vi "Main.vi"() -> ()   [LabVIEW 2017]
uses:
  LabVIEW/Controls/Recording Settings.ctl
  LabVIEW/Controls/Probe Dimensions.ctl
  LabVIEW/Controls/Rigid Body Info.ctl
  LabVIEW/Controls/Position.ctl
  LabVIEW/Controls/Orientation.ctl
  LabVIEW/Controls/Room Dimensions.ctl
  LabVIEW/Controls/Refnums.ctl
  <vilib>/userdefined/High Color/IMAQdx.ctl
  LabVIEW/Controls/Tracker Type.ctl
  LabVIEW/Controls/COM Port.ctl
  LabVIEW/Controls/Frame Grabber State.ctl
  LabVIEW/Controls/Optitrack State.ctl
  LabVIEW/Controls/Enabled State Control.ctl
  LabVIEW/Controls/Frame Grabber Data.ctl
  <vilib>/vision/Image Controls.llb/IMAQ Image.ctl
  <vilib>/vision/Avi.llb/IMAQ AVI2 Refnum.ctl
panel:
  out "Time (s)":dbl
  in  "Gestation":string
  in  "Connection Settings":T4={"Frame Grabber"="cam1", "Tracker"=enum."Aurora", "Port"=enum."COM1"} caption="These settings must be set BEFORE running the program!"
  in  "Refnums":T5
  out "Tracked?":bool
  out "Crop ROI":i32[](array[numeric])
  in  "Clear Crop":bool
  in  "Append":bool
  in  "Presentation":string
  in  "Crop":bool
  in  "Pause":bool
  out "Video Playback Filename":path
  in  "Frame Slider":u32(slide) scale=0.0..1138.0
  in  "Playback":bool
  in  "Room Dimensions":T6={"Room Width"=1000.0, "Room Depth"=1000.0, "Room Height"=1000.0}
  in  "Home":bool
  in  "Probe Dimensions":T7={"Probe Width"=50.0, "Probe Depth"=75.0, "Probe Height"=100.0} {"Probe Height" min=0.001; "Probe Depth" min=0.001; "Probe Width" min=0.001}
  in  "Recording Settings":T8={"Folder to Save Recording"=path "C:/Users/lydia/Desktop/Images", "Recording Name"="Test", "Video FPS"=5.0, "Codec"=3, "Operator"=0, "Tracker FPS"=40.0} {"Tracker FPS" min=1.0 max=100.0 format="%_6g"; "Operator" items=["Novice", "Expert"]; "Codec" items=["Cinepak Codec by Radius", "Intel IYUV codec", "Microsoft Video 1", "FF Video Codec 1 (FFV1) (NI Vision)", "Motion JPEG (NI Vision)", "Y800 Uncompressed Grey Scale (NI Vision)", "YUV 4:2:0 Planar (NI Vision)"]; "Video FPS" min=0.01 max=100.0 format="%.4f"}
  in  "Record":bool
  out "Tracker \nConnected?":bool
  out "Frame Grabber \nConnected?":bool
  out "Ultrasound Image":T9(plugin-control)
  in  "Live":bool
  in  "stop":bool
  in  "Probe Position":enum32{"3D", "Data"}(tab)
  out "Probe Position":refnum<vi>(3d-picture)
  out "Rigid Body":T10 caption="Probe Position Data"
  # "Frame"
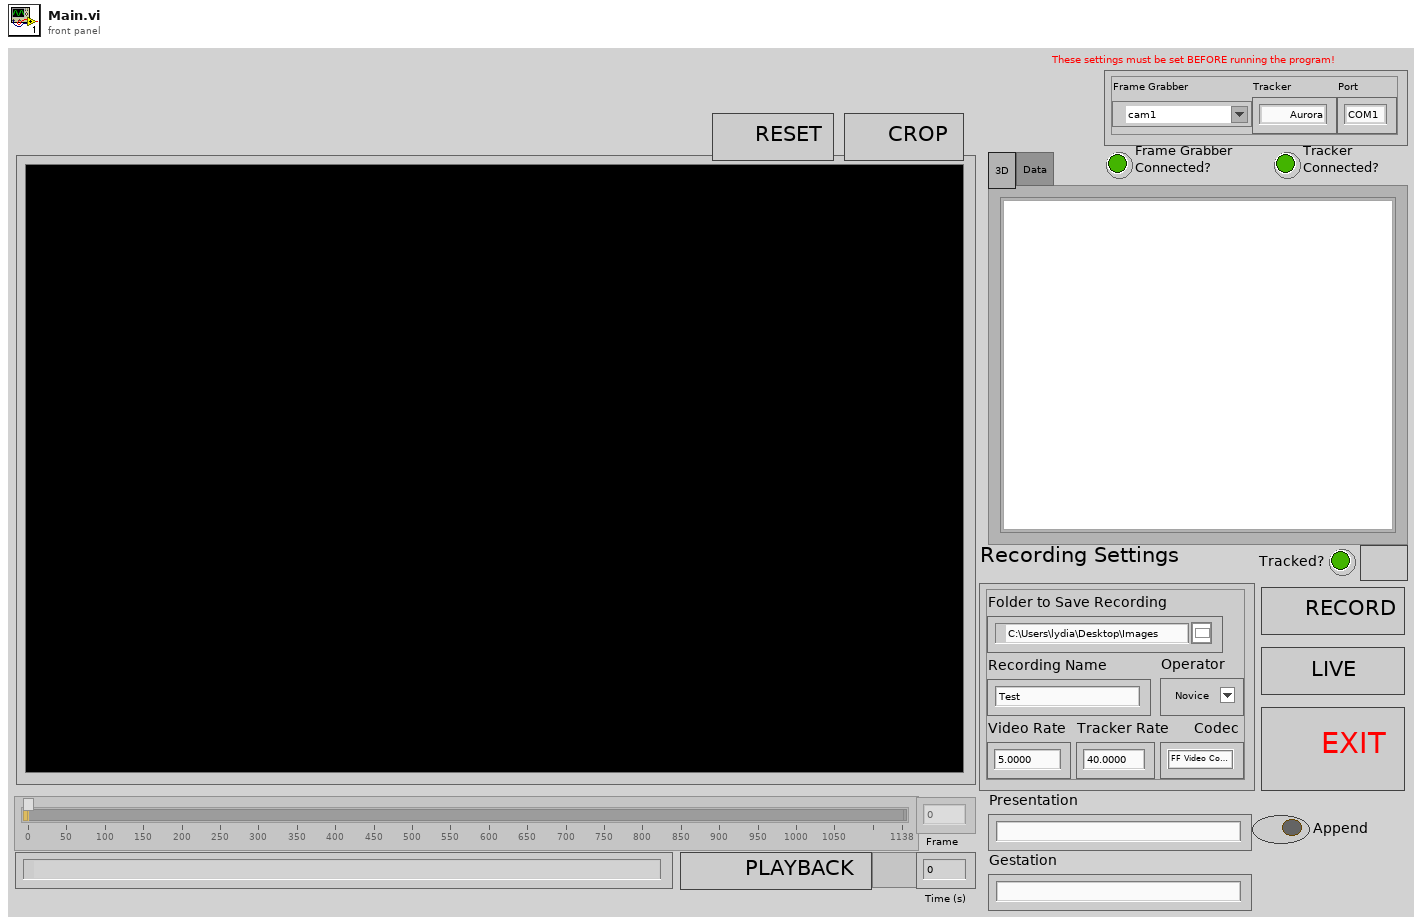
[diagram p1: front panel]
types:
  T1 = typedef "IMAQdx.ctl" = refnum<k21>
  T2 = typedef "Tracker Type.ctl" = enum16{"Aurora", "OptiTrack"}
  T3 = typedef "COM Port.ctl" = enum16{"COM1", "COM2", "COM3", "COM4", "COM5", "COM6", "COM7", "COM8", "COM9"}
  T4 = cluster{"Frame Grabber":T1, "Tracker":T2, "Port":T3}
  T5 = typedef "Refnums.ctl" = cluster{"Live Refnum":refnum<vi>, "Record Refnum":refnum<vi>, "Recording Settings Refnum":refnum<vi>, "Playback Refnum":refnum<vi>, "Frame Slider Refnum":refnum<vi>, "Pause Refnum":refnum<vi>, "Home Refnum":refnum<vi>, "Crop Refnum":refnum<vi>, "Clear Crop Refnum":refnum<vi>, "Connection Settings Refnum":refnum<vi>, "stop refnum":refnum<vi>}
  T6 = typedef "Room Dimensions.ctl" = cluster{"Room Width":dbl, "Room Depth":dbl, "Room Height":dbl}
  T7 = typedef "Probe Dimensions.ctl" = cluster{"Probe Width":sgl, "Probe Depth":sgl, "Probe Height":sgl}
  T8 = typedef "Recording Settings.ctl" = cluster{"Folder to Save Recording":path, "Recording Name":string, "Video FPS":dbl, "Codec":u16, "Operator":u16, "Tracker FPS":dbl}
  T9 = typedef "IMAQ Image.ctl" = refnum<image>
  T10 = typedef "Rigid Body Info.ctl" = cluster{"Position":T11, "Orientation":T12, "Quaternion":cluster{"qx":sgl, "qy":sgl, "qz":sgl, "qw":sgl}, "Tracked?":bool}
  T11 = typedef "Position.ctl" = cluster{"x (mm)":sgl, "y (mm)":sgl, "z (mm)":sgl}
  T12 = typedef "Orientation.ctl" = cluster{"Pitch (rad)":sgl, "Yaw (rad)":sgl, "Roll (rad)":sgl}
  T13 = typedef "Enabled State Control.ctl" = enum16{"Wait", "Start Live", "Start Recording", "Start Playback", "Shutdown"}
  T14 = typedef "Optitrack State.ctl" = enum16{"Wait", "Init", "Grab Rigid Body Data", "Error Handling", "Shutdown"}
  T15 = typedef "Frame Grabber State.ctl" = enum16{"Wait", "Init", "Update Geometry", "Set Crop ROI", "Clear Crop ROI", "Configure Live", "Configure Recording", "Start Playback", "Grab Live Frame", "Record Frame", "Playback Frame", "Unconfigure Live", "End Recording", "Stop Playback", "Error Handling", "Shutdown"}
  T16 = typedef "Queues.ctl" = cluster{"Frame Grabber State":refnum<queue>, "Tracker State":refnum<queue>}
  T17 = typedef "Frame Grabber Data.ctl" = cluster{"Camera Session":T1, "Frame":T9, "AVI Refnum":T18, "Codecs":string[], "Frame number":u32, "Tracking File Refnum":refnum<file>, "Tick Count":u32, "Probe Object":refnum<vi>, "Playback Probe Data":dbl[][], "Rigid Body":T10, "Total no frames playback":u32, "Playback Video FPS":u32, "Camera connected?":bool, "Scene":refnum<vi>, "Frame Number Refnum":refnum<vi>, "Cropped Frame":T9, "Playback Tracker FPS":u32, "Crop ROI":i32[], "Presentation Values":string[], "Elapsed time (ms)":u32, "Camera frames playback":u32, "Gestation":string}
  T18 = typedef "IMAQ AVI2 Refnum.ctl" = refnum<k20>
  T19 = enum8{"Enabled", "Disabled", "Disabled and Grayed Out"}
  T20 = typedef "Tracking Data.ctl" = cluster{"VISA resource name":refnum<visa-resource-name>, "Packet Data":T21, "Rigid Body Data":T10, "Position Array":dbl[][], "Tracker":T2}
  T21 = typedef "Packet Data.ctl" = cluster{"Frame Number (UINT32)":u32, "Number of Rigid Bodies (UINT32)":u32, "Timestamp (double float)":dbl}
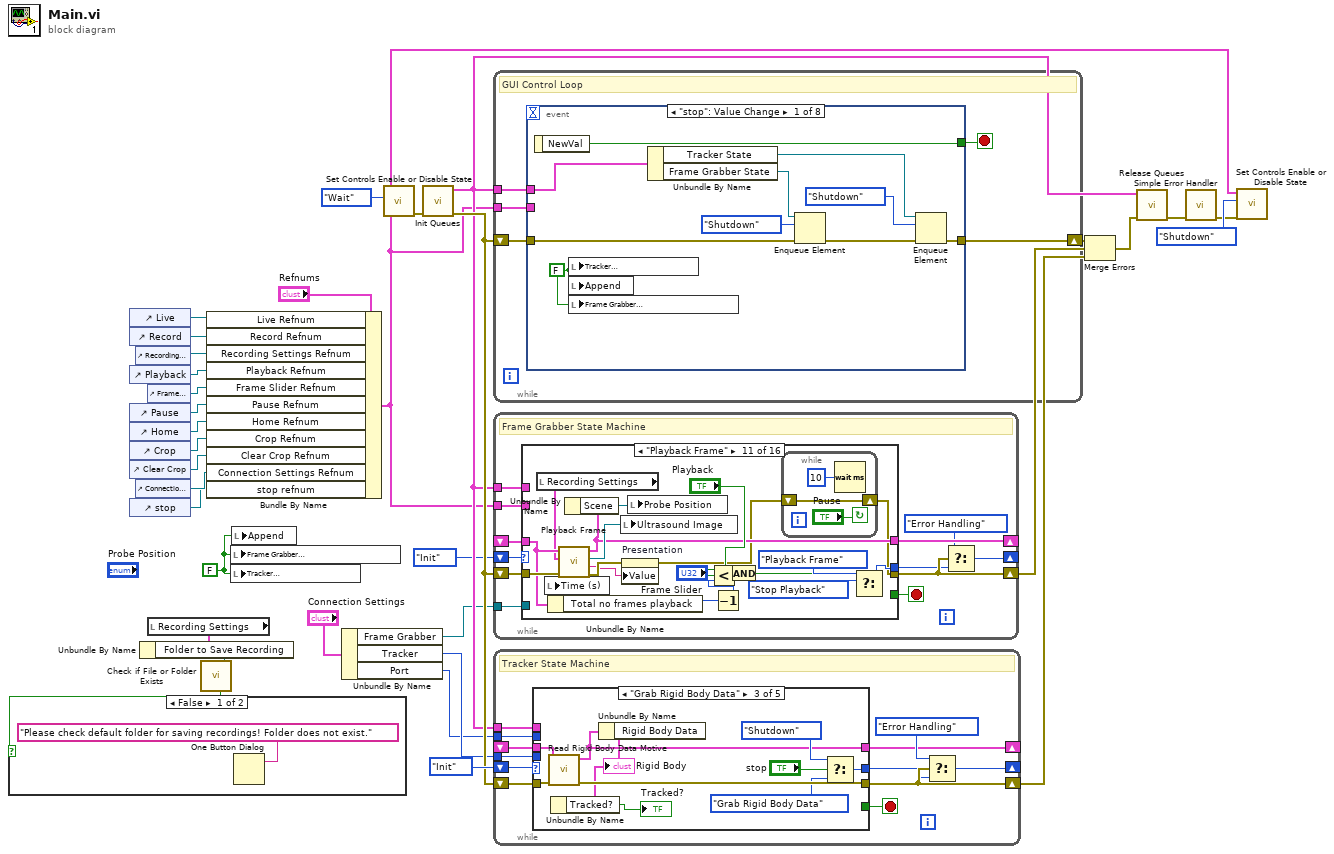
[diagram p0: block diagram]
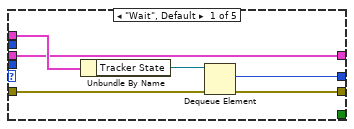
[diagram p3: hidden frame]
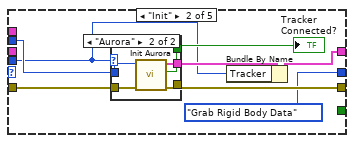
[diagram p4: hidden frame]
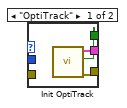
[diagram p5: hidden frame]
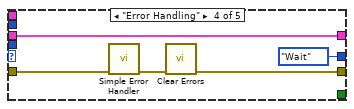
[diagram p6: hidden frame]
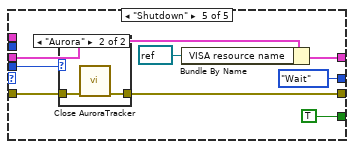
[diagram p7: hidden frame]
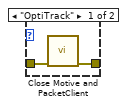
[diagram p8: hidden frame]
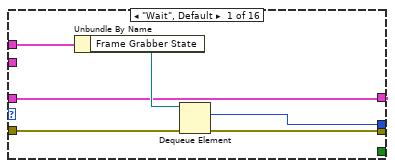
[diagram p9: hidden frame]
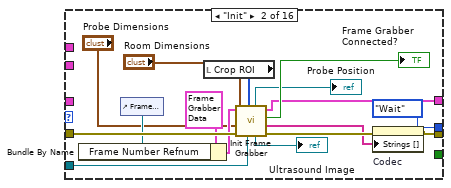
[diagram p10: hidden frame]
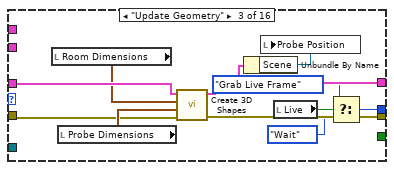
[diagram p11: hidden frame]
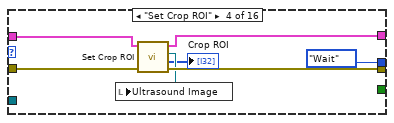
[diagram p12: hidden frame]
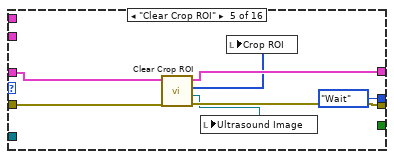
[diagram p13: hidden frame]
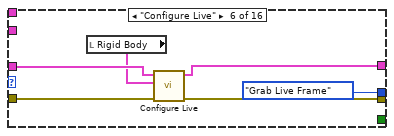
[diagram p14: hidden frame]
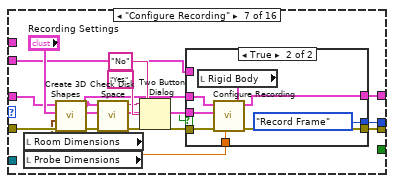
[diagram p15: hidden frame]
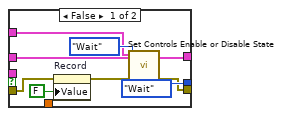
[diagram p16: hidden frame]
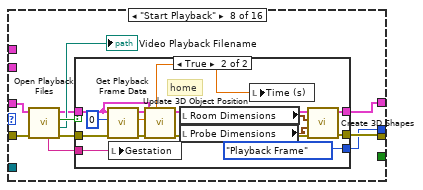
[diagram p17: hidden frame]
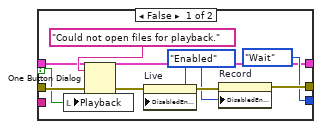
[diagram p18: hidden frame]
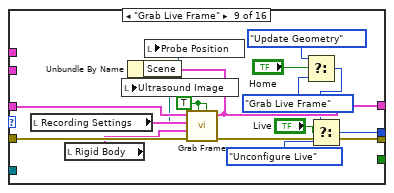
[diagram p19: hidden frame]
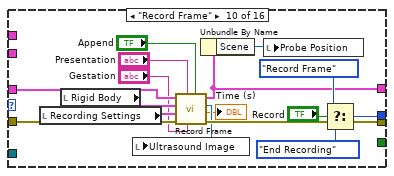
[diagram p20: hidden frame]
diagram:
  w13 = FALSE ("Camera Connected?")
  n1 = control-ref of="Live"() -> (w25:refnum<vi>)
  n2 = control-ref of="Record"() -> (w24:refnum<vi>)
  n3 = control-ref of="Playback"() -> (w22:refnum<vi>)
  n4 = control-ref of="Pause"() -> (w20:refnum<vi>)
  n5 = control-ref of="Home"() -> (w19:refnum<vi>)
  n6 = control-ref of="Crop"() -> (w18:refnum<vi>)
  n7 = control-ref of="Clear Crop"() -> (w17:refnum<vi>)
  n8 = control-ref of="stop"() -> (w1:refnum<vi>)
  n9 = control-ref of="Recording Settings"() -> (w23:refnum<vi>)
  n10 = control-ref of="Connection Settings"() -> (w2:refnum<vi>)
  n11 = control-ref of="Frame Slider"() -> (w21:refnum<vi>)
  n12 = local read "Recording Settings"() -> (w12:T8)
  n13 = Unbundle By Name(w12) -> ("Folder to Save Recording"=w11:path)
  n14 = call <vilib>:"Check if File or Folder Exists.vi"("path"=w11) -> ("file or folder exists?"=w10:bool)  [unwired: 8 in, 2 out]
  n15 = case shown="False" w10 {
    frame False {
      n16 = One Button Dialog(message="Please check default folder for saving recordings! Folder does not exist.") -> ()  [unwired: 1 in, 1 out]
    }
    frame True {
    }
  }
  n17 = Bundle By Name(cluster="Refnums", "Live Refnum"=w25, "Record Refnum"=w24, "Recording Settings Refnum"=w23, "Playback Refnum"=w22, "Frame Slider Refnum"=w21, "Pause Refnum"=w20, "Home Refnum"=w19, "Crop Refnum"=w18, "Clear Crop Refnum"=w17, "Connection Settings Refnum"=w2, "stop refnum"=w1) -> (w7:T5)
  n18 = local write "Frame Grabber \nConnected?"(w13) -> ()
  n19 = local write "Tracker \nConnected?"(w13) -> ()
  n20 = local write "Append"(w13) -> ()
  n21 = Unbundle By Name("Connection Settings") -> ("Frame Grabber"=w5:T1, "Tracker"=w4:T2, "Port"=w3:T3)
  n22 = call "Set Controls Enable or Disable State.vi"("Refnum State"=Enabled_State_Control."Wait", "Refnums In"=w7) -> ("error out"=w15:errorcluster)  [unwired: 9 in]
  n23 = call "Init Queues.vi"("error in (no error) in"=w15) -> ("error out"=w29:errorcluster, "Queues"=w28:T16)  [unwired: 9 in]
  n24 = while {
    shift-right: [w38] -> w34
    shift-left: w29 -> [w39]
    tunnel: w28 -> [w37]
    tunnel: w7 -> [w36]
    stop <- w40 stop-if-true
    # "GUI Control Loop"
    n25 = event shown="[0] \"stop\": Value Change" {
      selector: _ -> [_ _ _ _ _ _ _ _]
      dyn-events: _ -> [_ _ _ _ _ _ _ _]
      timeout: _ -> [_ _ _ _ _ _ _ _]
      tunnel: [w43 _ _ _ _ _ _ _] -> w40
      tunnel: w39 -> [w42 w63 w77 w79 w87 w92 w105 w106]
      tunnel: [w46 w56 w68 w78 w83 w88 w96 w106] -> w38
      tunnel: w37 -> [w50 w60 w74 w82 w86 w91 w102 _]
      tunnel: w36 -> [_ w55 w70 _ _ _ w98 _]
      event "stop": Value Change {
        w41 = FALSE ("Run")
        n26 = event-data() -> ("NewVal"=w43:bool)  [unwired: 1 in]
        n27 = local write "Tracker \nConnected?"(w41) -> ()
        n28 = local write "Append"(w41) -> ()
        n29 = local write "Frame Grabber \nConnected?"(w41) -> ()
        n30 = Unbundle By Name(w50) -> ("Tracker State"=w45:refnum<queue>, "Frame Grabber State"=w49:refnum<queue>)
        n31 = Enqueue Element(queue=w49, element=Frame_Grabber_State."Shutdown", error in (no error)=w42) -> (error out=w47:errorcluster)  [unwired: 1 in, 2 out]
        n32 = Enqueue Element(queue=w45, element=Optitrack_State."Shutdown", error in (no error)=w47) -> (error out=w46:errorcluster)  [unwired: 1 in, 2 out]
      }
      event "Live": Value Change {
        n33 = event-data() -> ("NewVal"=w52:bool)  [unwired: 1 in]
        n34 = Unbundle By Name(w60) -> ("Frame Grabber State"=w59:refnum<queue>)
        n35 = Select(t=Frame_Grabber_State."Configure Live", s=w52, f=Frame_Grabber_State."Wait") -> (s? t:f=w61:T15)
        n36 = Enqueue Element(queue=w59, element=w61, error in (no error)=w63) -> (error out=w57:errorcluster)  [unwired: 1 in, 2 out]
        n37 = Select(t=Enabled_State_Control."Start Live" ("Refnum State"), s=w52, f=Enabled_State_Control."Wait") -> (s? t:f=w53:T13)
        n38 = call "Set Controls Enable or Disable State.vi"("error in (no error)"=w57, "Refnum State"=w53, "Refnums In"=w55) -> ("error out"=w56:errorcluster)  [unwired: 8 in]
      }
      event "Playback": Value Change {
        n39 = event-data() -> ("NewVal"=w66:bool)  [unwired: 1 in]
        n40 = Unbundle By Name(w74) -> ("Frame Grabber State"=w73:refnum<queue>)
        n41 = Select(t=Frame_Grabber_State."Start Playback", s=w66, f=Frame_Grabber_State."Wait") -> (s? t:f=w75:T15)
        n42 = Enqueue Element(queue=w73, element=w75, error in (no error)=w77) -> (error out=w69:errorcluster)  [unwired: 1 in, 2 out]
        n43 = Select(t=Enabled_State_Control."Start Playback", s=w66, f=Enabled_State_Control."Wait" ("Refnum State")) -> (s? t:f=w65:T13)
        n44 = local write "Pause"(FALSE ("Pause")) -> ()
        n45 = call "Set Controls Enable or Disable State.vi"("error in (no error)"=w69, "Refnum State"=w65, "Refnums In"=w70) -> ("error out"=w68:errorcluster)  [unwired: 8 in]
      }
      event "Home": Value Change {
        n46 = event-data() -> ()  [unwired: 1 in, 4 out]
        n47 = Unbundle By Name(w82) -> ("Frame Grabber State"=w81:refnum<queue>)
        n48 = Enqueue Element(queue=w81, element=Frame_Grabber_State."Update Geometry", error in (no error)=w79) -> (error out=w78:errorcluster)  [unwired: 1 in, 2 out]
      }
      event "Crop": Value Change {
        n49 = event-data() -> ()  [unwired: 1 in, 4 out]
        n50 = Unbundle By Name(w86) -> ("Frame Grabber State"=w85:refnum<queue>)
        n51 = Enqueue Element(queue=w85, element=Frame_Grabber_State."Set Crop ROI", error in (no error)=w87) -> (error out=w83:errorcluster)  [unwired: 1 in, 2 out]
      }
      event "Clear Crop": Value Change {
        n52 = event-data() -> ()  [unwired: 1 in, 4 out]
        n53 = Unbundle By Name(w91) -> ("Frame Grabber State"=w90:refnum<queue>)
        n54 = Enqueue Element(queue=w90, element=Frame_Grabber_State."Clear Crop ROI", error in (no error)=w92) -> (error out=w88:errorcluster)  [unwired: 1 in, 2 out]
      }
      event "Record": Value Change {
        n55 = event-data() -> ("NewVal"=w99:bool)  [unwired: 1 in]
        n56 = Unbundle By Name(w102) -> ("Frame Grabber State"=w101:refnum<queue>)
        n57 = Select(t=Frame_Grabber_State."Configure Recording", s=w99, f=Frame_Grabber_State."Wait") -> (s? t:f=w103:T15)
        n58 = Enqueue Element(queue=w101, element=w103, error in (no error)=w105) -> (error out=w97:errorcluster)  [unwired: 1 in, 2 out]
        n59 = Select(t=Enabled_State_Control."Start Recording" ("Refnum State"), s=w99, f=Enabled_State_Control."Wait" ("Refnum State")) -> (s? t:f=w93:T13)
        n60 = call "Set Controls Enable or Disable State.vi"("error in (no error)"=w97, "Refnum State"=w93, "Refnums In"=w98) -> ("error out"=w96:errorcluster)  [unwired: 8 in]
      }
      event "Presentation": Value Change {
        n61 = event-data() -> ()  [unwired: 1 in, 1 out]
        n62 = local write "Append"(TRUE ("Append")) -> ()
      }
    }
  }
  n63 = while {
    shift-right: [w111] -> _
    shift-left: Frame_Grabber_State."Init" -> [w119]
    shift-right: [w113] -> w33
    shift-left: w29 -> [w118]
    tunnel: w28 -> [w117]
    shift-right: [w115] -> _
    shift-left: _ -> [w114]
    tunnel: w7 -> [w109]
    tunnel: w5 -> [w108]
    stop <- w116 stop-if-true
    # "Frame Grabber State Machine"
    n64 = case shown="\"Playback Frame\"" w119 {
      tunnel: w118 -> [w125 w141 w150 w158 w164 w172 w178 w215 w253 w265 w286 w296 w300 w311 w317 w326]
      tunnel: [w124 w137 w149 w157 w163 w171 w187 w212 w252 w264 w276 w294 w297 w304 w314 w325] -> w113
      tunnel: w117 -> [w123 _ _ _ _ _ _ _ _ _ _ _ _ _ _ _]
      tunnel: [w121 Frame_Grabber_State."Wait" w143 Frame_Grabber_State."Wait" Frame_Grabber_State."Wait" Frame_Grabber_State."Grab Live Frame" w189 w211 w250 w267 w288 Frame_Grabber_State."Wait" Frame_Grabber_State."Wait" Frame_Grabber_State."Wait" Frame_Grabber_State."Wait" Frame_Grabber_State."Wait"] -> w112
      tunnel: [_ _ _ _ _ _ _ _ _ _ _ _ _ _ _ TRUE] -> w116
      tunnel: [w120 w129 w148 w155 w162 w168 w188 w206 w245 w258 w278 w293 w298 w308 w318 w323] -> w115
      tunnel: w114 -> [w120 _ w152 w156 w165 w170 w176 w214 w248 w261 w280 w293 w298 w309 w318 w324]
      tunnel: w109 -> [_ _ _ _ _ _ w179 _ _ _ _ _ _ w301 w313 _]
      tunnel: w108 -> [_ w126 _ _ _ _ _ _ _ _ _ _ _ _ _ _]
      frame "Wait", Default {
        n65 = Unbundle By Name(w123) -> ("Frame Grabber State"=w122:refnum<queue>)
        n66 = Dequeue Element(queue=w122, error in (no error)=w125) -> (element=w121:T15, error out=w124:errorcluster)  [unwired: 1 in, 2 out]
      }
      frame "Init" {
        n67 = control-ref of="Frame Slider"() -> (w134:refnum<vi>)
        n68 = Bundle By Name(cluster=T17 {"Camera Session"="", "Frame"=refnum, "AVI Refnum"=refnum, "Codecs"=[], "Frame number"=0, "Tracking File Refnum"=refnum, "Tick Count"=0, "Probe Object"=refnum, "Playback Probe Data"=[], "Rigid Body"={"Position"={"x (mm)"=0.0, "y (mm)"=0.0, "z (mm)"=0.0}, "Orientation"={"Pitch (rad)"=0.0, "Yaw (rad)"=0.0, "Roll (rad)"=0.0}, "Quaternion"={"qx"=0.0, "qy"=0.0, "qz"=0.0, "qw"=0.0}, "Tracked?"=FALSE}, "Total no frames playback"=0, "Playback Video FPS"=0, "Camera connected?"=FALSE, "Scene"=refnum, "Frame Number Refnum"=refnum, "Cropped Frame"=refnum, "Playback Tracker FPS"=0, "Crop ROI"=[], "Presentation Values"=[], "Elapsed time (ms)"=0, "Camera frames playback"=0, "Gestation"=""} ("Frame Grabber Data"), "Frame Number Refnum"=w134) -> (w133:T17)
        n69 = local read "Crop ROI"() -> (w127:i32[])
        n70 = call "Init Frame Grabber.vi"("Frane Grabber"=w126, "Crop ROI Rectangle"=w127, "Error In"=w141, "Probe Dimensions"="Probe Dimensions", "Room Dimensions"="Room Dimensions", "Frame Grabber Data"=w133) -> ("Error Out"=w138:errorcluster, "Codec Names"=w136:string[], "Frame Grabber Connected?"=→"Frame Grabber \nConnected?":bool, "Frame Grabber Data Out"=w129:T17, "Image Out"=→"Ultrasound Image":T9, "Scene"=→"Probe Position":refnum<vi>)
        n71 = property on="Codec" class="Ring (strict)"(error in=w138, "Strings []"=w136) -> (error out=w137:errorcluster)  [unwired: 1 in, 1 out]
      }
      frame "Update Geometry" {
        n72 = local read "Room Dimensions"() -> (w142:T6)
        n73 = local read "Probe Dimensions"() -> (w151:T7)
        n74 = call "Create 3D Shapes.vi"("error in (no error)"=w150, "Probe Dimensions"=w151, "Room Dimensions"=w142, "Frame Grabber Data In"=w152) -> ("error out"=w149:errorcluster, "Frame Grabber Data Out"=w148:T17)  [unwired: 6 in]
        n75 = Unbundle By Name(w148) -> ("Scene"=w147:refnum<vi>)
        n76 = local write "Probe Position"(w147) -> ()
        n77 = local read "Live"() -> (w146:bool)
        n78 = Select(t=Frame_Grabber_State."Grab Live Frame", s=w146, f=Frame_Grabber_State."Wait") -> (s? t:f=w143:T15)
      }
      frame "Set Crop ROI" {
        n79 = call "Set Crop ROI.vi"("error in (no error)"=w158, "Frame Grabber Data in"=w156) -> ("error out"=w157:errorcluster, "Crop ROI"=→"Crop ROI":i32[], "Image Out"=w154:T9, "Frame Grabber Data out"=w155:T17)  [unwired: 6 in]
        n80 = local write "Ultrasound Image"(w154) -> ()
      }
      frame "Clear Crop ROI" {
        n81 = call "Clear Crop ROI.vi"("error in (no error)"=w164, "Frame Grabber Data in"=w165) -> ("error out"=w163:errorcluster, "Image Out"=w161:T9, "Crop ROI"=w160:i32[], "Frame Grabber Data out"=w162:T17)  [unwired: 6 in]
        n82 = local write "Ultrasound Image"(w161) -> ()
        n83 = local write "Crop ROI"(w160) -> ()
      }
      frame "Configure Live" {
        n84 = local read "Rigid Body"() -> (w167:T10)
        n85 = call "Configure Live.vi"("error in (no error)"=w172, "Rigid Body"=w167, "Frame Grabber Data in"=w170) -> ("error out"=w171:errorcluster, "Frame Grabber Data out"=w168:T17)  [unwired: 7 in]
      }
      frame "Configure Recording" {
        n86 = local read "Room Dimensions"() -> (w173:T6)
        n87 = local read "Probe Dimensions"() -> (w174:T7)
        n88 = call "Create 3D Shapes.vi"("error in (no error)"=w178, "Probe Dimensions"=w174, "Room Dimensions"=w173, "Frame Grabber Data In"=w176) -> ("error out"=w177:errorcluster, "Frame Grabber Data Out"=w175:T17)  [unwired: 6 in]
        n89 = call "Check Disk Space.vi"("Error In"=w177, "Recording Settings"="Recording Settings", "Frame Grabber Data"=w175) -> ("Error Out"=w182:errorcluster, "Max number of frames"=w180:dbl, "Prompt"=w181:string)  [unwired: 5 in, 1 out]
        n90 = Two Button Dialog(message=w181, 1:"No" ("F button name (\"Cancel\")"), 2:"Yes" ("T button name (\"OK\")")) -> (T button?=w183:bool)
        n91 = case shown="True" w183 {
          tunnel: [Frame_Grabber_State."Wait" Frame_Grabber_State."Record Frame"] -> w189
          tunnel: [w197 w204] -> w188
          tunnel: [w192 w203] -> w187
          tunnel: "Recording Settings" -> [_ w201]
          tunnel: w175 -> [w197 w200]
          tunnel: w182 -> [w194 w199]
          tunnel: w180 -> [_ w198]
          tunnel: w179 -> [w190 _]
          frame False {
            n92 = property on="Record" class="Bool (strict)"(error in=w194, "Value"=FALSE ("Record")) -> (error out=w193:errorcluster)  [unwired: 1 in, 1 out]
            n93 = call "Set Controls Enable or Disable State.vi"("error in (no error)"=w193, "Refnum State"=Enabled_State_Control."Wait", "Refnums In"=w190) -> ("error out"=w192:errorcluster)  [unwired: 8 in]
          }
          frame True {
            n94 = local read "Rigid Body"() -> (w202:T10)
            n95 = call "Configure Recording.vi"("Max number of frames"=w198, "error in (no error)"=w199, "Rigid Body"=w202, "Recording Settings"=w201, "Frame Grabber Data In"=w200) -> ("error out"=w203:errorcluster, "Frame Grabber Data Out"=w204:T17)  [unwired: 5 in]
          }
        }
      }
      frame "Start Playback" {
        n96 = call "Open Playback Files.vi"("error in (no error)"=w215, "Frame Grabber Data In"=w214) -> ("error out"=w213:errorcluster, "Playback Video"=→"Video Playback Filename":path, "both exist and open?"=w210:bool, "Frame Grabber Data Out"=w207:T17, "Gestation"=w208:string)  [unwired: 5 in]
        n97 = case shown="True" w210 {
          selector: w210 -> [w217 _]
          tunnel: w213 -> [w221 w235]
          tunnel: [w220 w234] -> w212
          tunnel: [Frame_Grabber_State."Wait" ("f") Frame_Grabber_State."Playback Frame"] -> w211
          tunnel: w208 -> [_ w236]
          tunnel: w207 -> [w216 w228]
          tunnel: [w216 w230] -> w206
          frame False {
            w218 = T19."Enabled" ("Disabled")
            n98 = local write "Playback"(w217) -> ()
            n99 = One Button Dialog(message="Could not open files for playback.") -> ()  [unwired: 1 in, 1 out]
            n100 = property on="Live" class="Bool (strict)"(error in=w221, "DisabledEnum"=w218) -> (error out=w222:errorcluster)  [unwired: 1 in, 1 out]
            n101 = property on="Record" class="Bool (strict)"(error in=w222, "DisabledEnum"=w218) -> (error out=w220:errorcluster)  [unwired: 1 in, 1 out]
          }
          frame True {
            # "home"
            n102 = call "Get Playback Frame Data.vi"("Error In"=w235, "Frame number"=u32 0, "Frame Grabber Data"=w228) -> ("Error Out"=w227:errorcluster, "Time elapsed (s)"=w232:dbl, "New Rigid Body Position"=w229:T10)  [unwired: 4 in, 2 out]
            n103 = local write "Gestation"(w236) -> ()
            n104 = call "Update 3D Object Position.vi"("error in (no error)"=w227, "New Rigid Body Position"=w229, "Frame Grabber Data in"=w228) -> ("error out"=w231:errorcluster, "Frame Grabber Data out"=w226:T17)  [unwired: 7 in]
            n105 = local read "Room Dimensions"() -> (w225:T6)
            n106 = local read "Probe Dimensions"() -> (w224:T7)
            n107 = local write "Time (s)"(w232) -> ()
            n108 = call "Create 3D Shapes.vi"("error in (no error)"=w231, "Probe Dimensions"=w224, "Room Dimensions"=w225, "Frame Grabber Data In"=w226) -> ("error out"=w234:errorcluster, "Frame Grabber Data Out"=w230:T17)  [unwired: 6 in]
          }
        }
      }
      frame "Grab Live Frame" {
        w239 = TRUE
        n109 = local read "Recording Settings"() -> (w249:T8)
        n110 = local read "Rigid Body"() -> (w247:T10)
        n111 = call "Grab Frame.vi"("Live?"=w239, "Grab frame?"=w239, "error in (no error)"=w253, "Rigid Body"=w247, "Recording Settings"=w249, "Frame Grabber Data in"=w248) -> ("error out"=w252:errorcluster, "Frame"=w238:T9, "Frame Grabber Data out"=w245:T17)  [unwired: 2 in, 1 out]
        n112 = local write "Ultrasound Image"(w238) -> ()
        n113 = Unbundle By Name(w245) -> ("Scene"=w246:refnum<vi>)
        n114 = local write "Probe Position"(w246) -> ()
        n115 = Select(t=Frame_Grabber_State."Update Geometry", s="Home", f=Frame_Grabber_State."Grab Live Frame") -> (s? t:f=w241:T15)
        n116 = Select(t=w241, s="Live", f=Frame_Grabber_State."Unconfigure Live") -> (s? t:f=w250:T15)
      }
      frame "Record Frame" {
        n117 = local read "Recording Settings"() -> (w260:T8)
        n118 = local read "Rigid Body"() -> (w263:T10)
        n119 = call "Record Frame.vi"("Append"="Append", "Gestation"="Gestation", "Presentation"="Presentation", "error in (no error)"=w265, "Recording Settings"=w260, "Probe Position"=w263, "Frame Grabber Data In in"=w261) -> ("error out"=w264:errorcluster, "Time elapsed (s)"=→"Time (s)":dbl, "Image"=w262:T9, "Frame Grabber Data out"=w258:T17)  [unwired: 1 in]
        n120 = local write "Ultrasound Image"(w262) -> ()
        n121 = Unbundle By Name(w258) -> ("Scene"=w259:refnum<vi>)
        n122 = local write "Probe Position"(w259) -> ()
        n123 = Select(t=Frame_Grabber_State."Record Frame", s="Record", f=Frame_Grabber_State."End Recording") -> (s? t:f=w267:T15)
      }
      frame "Playback Frame" {
        n124 = local read "Recording Settings"() -> (w277:T8)
        n125 = Unbundle By Name(w280) -> ("Total no frames playback"=w283:u32)
        n126 = call "Playback Frame.vi"("error in (no error)"=w286, "Recording Settings"=w277, "Frame Grabber Data in"=w280) -> ("error out"=w273:errorcluster, "Presentation"=w271:string, "Image"=w285:T9, "Frame Grabber Data out"=w278:T17, "Time elapsed (s)"=w270:dbl)  [unwired: 4 in]
        n127 = local write "Time (s)"(w270) -> ()
        n128 = Unbundle By Name(w278) -> ("Scene"=w275:refnum<vi>)
        n129 = local write "Ultrasound Image"(w285) -> ()
        n130 = property on="Presentation" class="Str"(error in=w273, "Value"=w271) -> (error out=w272:errorcluster)  [unwired: 1 in, 1 out]
        n131 = local write "Probe Position"(w275) -> ()
        n132 = Decrement(x=w283) -> (x-1=w274:u32)
        n133 = Less?(x="Frame Slider", y=w274) -> (x < y?=w284:bool)
        n134 = And(x=w284, y="Playback") -> (x .and. y?=w282:bool)
        n135 = while {
          shift-right: [w290] -> w276
          shift-left: w272 -> [w290]
          stop <- "Pause" continue-if-true
          n136 = Wait (ms)(milliseconds to wait=u32 10) -> ()  [unwired: 1 out]
        }
        n137 = Select(t=Frame_Grabber_State."Playback Frame", s=w282, f=Frame_Grabber_State."Stop Playback") -> (s? t:f=w288:T15)
      }
      frame "Unconfigure Live" {
        n138 = call "Unconfigure Live.vi"("error in (no error)"=w296, "Frame Grabber Data in"=w293) -> ("error out"=w294:errorcluster)  [unwired: 9 in]
      }
      frame "End Recording" {
        n139 = call "End Recording.vi"("error in (no error)"=w300, "Frame Grabber Data in"=w298) -> ("error out"=w297:errorcluster)  [unwired: 9 in]
      }
      frame "Stop Playback" {
        n140 = Unbundle By Name(w309) -> ("AVI Refnum"=w310:T18)
        n141 = call "IMAQ AVI2 Close"("error in (no error)"=w311, "AVI Refnum"=w310) -> ("error out"=w305:errorcluster)  [unwired: 9 in]
        n142 = local write "Playback"(FALSE ("Playback")) -> ()
        n143 = call "Set Controls Enable or Disable State.vi"("error in (no error)"=w305, "Refnum State"=Enabled_State_Control."Wait", "Refnums In"=w301) -> ("error out"=w304:errorcluster)  [unwired: 8 in]
        n144 = Bundle By Name(cluster=w309, "AVI Refnum"=refnum<k0> refnum) -> (w308:T17)
      }
      frame "Error Handling" {
        # "just in case"
        n145 = call "End Recording.vi"("error in (no error)"=w317, "Frame Grabber Data in"=w318) -> ("error out"=w316:errorcluster)  [unwired: 9 in]
        n146 = call <vilib>:"Simple Error Handler.vi"("error in (no error)"=w316) -> ("error out"=w320:errorcluster)  [unwired: 4 in, 4 out]
        n147 = call <vilib>:"Clear Errors.vi"("error in (no error)"=w320) -> ("error out"=w315:errorcluster)  [unwired: 5 in, 1 out]
        n148 = call "Set Controls Enable or Disable State.vi"("error in (no error)"=w315, "Refnum State"=Enabled_State_Control."Wait", "Refnums In"=w313) -> ("error out"=w314:errorcluster)  [unwired: 8 in]
      }
      frame "Shutdown" {
        n149 = local read "Frame Grabber \nConnected?"() -> (w321:bool)
        n150 = call "Shutdown Frame Grabber.vi"("error in (no error)"=w326, "Frame grabber connected?"=w321, "Frame Grabber Data in"=w324) -> ("error out"=w325:errorcluster, "Disconnect"=w322:bool, "Frame Grabber Data out"=w323:T17)  [unwired: 6 in]
        n151 = local write "Frame Grabber \nConnected?"(w322) -> ()
      }
    }
    n152 = Select(t=Frame_Grabber_State."Error Handling", s=w113, f=w112) -> (s? t:f=w111:T15)
  }
  n153 = while {
    shift-right: [w337] -> w26
    shift-left: w29 -> [w339]
    shift-right: [w335] -> _
    shift-left: Optitrack_State."Init" ("OptiTrack State") -> [w340]
    tunnel: w28 -> [w338]
    shift-right: [w332] -> _
    shift-left: _ -> [w331]
    tunnel: w4 -> [w330]
    tunnel: w3 -> [w329]
    stop <- w333 stop-if-true
    # "Tracker State Machine"
    n154 = case shown="\"Grab Rigid Body Data\"" w340 {
      tunnel: w339 -> [w346 w349 w372 w377 w384]
      tunnel: [w345 w353 w371 w375 w383] -> w337
      tunnel: w338 -> [w344 _ _ _ _]
      tunnel: [w343 Optitrack_State."Grab Rigid Body Data" ("OptiTrack State") w367 Optitrack_State."Wait" ("OptiTrack State") Optitrack_State."Wait" ("OptiTrack State")] -> w334
      tunnel: [_ _ _ _ TRUE] -> w333
      tunnel: [w342 w350 w366 w374 w380] -> w332
      tunnel: w331 -> [w342 _ w370 w374 w381]
      tunnel: w330 -> [_ w347 _ _ w378]
      tunnel: w329 -> [_ w348 _ _ _]
      frame "Wait", Default {
        n155 = Unbundle By Name(w344) -> ("Tracker State"=w341:refnum<queue>)
        n156 = Dequeue Element(queue=w341, error in (no error)=w346) -> (element=w343:T14, error out=w345:errorcluster)  [unwired: 1 in, 2 out]
      }
      frame "Init" {
        n157 = case shown="\"Aurora\"" w347 {
          tunnel: [w357 w362] -> w354
          tunnel: [w356 w361] -> w353
          tunnel: [w355 w360] -> w352
          tunnel: w349 -> [_ w359]
          tunnel: w348 -> [_ w358]
          frame "OptiTrack" {
            n158 = call "Init OptiTrack.vi"() -> ("error out"=w356:errorcluster, "OptiTrack Connected?"=w355:bool, "Frame Grabber Data"=w357:T20)  [unwired: 9 in]
          }
          frame "Aurora" {
            n159 = call "Init Aurora.vi"("error in (no error)"=w359, "Aurora COM Port"=w358) -> ("error out"=w361:errorcluster, "Aurora Connected?"=w360:bool, "Frame Grabber Data"=w362:T20)  [unwired: 7 in]
          }
        }
        "Tracker \nConnected?" <- w352
        n160 = Bundle By Name(cluster=w354, "Tracker"=w347) -> (w350:T20)
      }
      frame "Grab Rigid Body Data" {
        n161 = call "Read Rigid Body Data Motive.vi"("error in (no error)"=w372, "Tracking Data In"=w370) -> ("error out"=w371:errorcluster, "Tracking Data Out"=w366:T20)  [unwired: 8 in]
        n162 = Unbundle By Name(w366) -> ("Rigid Body Data"=w364:T10)
        "Rigid Body" <- w364
        n163 = Unbundle By Name(w364) -> ("Tracked?"=→"Tracked?":bool)
        n164 = Select(t=Optitrack_State."Shutdown" ("f"), s="stop", f=Optitrack_State."Grab Rigid Body Data" ("OptiTrack State")) -> (s? t:f=w367:T14)
      }
      frame "Error Handling" {
        n165 = call <vilib>:"Simple Error Handler.vi"("error in (no error)"=w377) -> ("error out"=w376:errorcluster)  [unwired: 4 in, 4 out]
        n166 = call <vilib>:"Clear Errors.vi"("error in (no error)"=w376) -> ("error out"=w375:errorcluster)  [unwired: 5 in, 1 out]
      }
      frame "Shutdown" {
        n167 = case shown="\"Aurora\"" w378 {
          tunnel: w384 -> [w387 w389]
          tunnel: [w386 w388] -> w383
          frame "OptiTrack" {
            n168 = call "Close Motive and PacketClient.vi"("Error In"=w387) -> ("Error Out"=w386:errorcluster)  [unwired: 10 in]
          }
          frame "Aurora" {
            n169 = call "Close AuroraTracker.vi"("Error In"=w389) -> ("Error Out"=w388:errorcluster)  [unwired: 10 in]
          }
        }
        n170 = Bundle By Name(cluster=w381, "VISA resource name"=refnum<visa-resource-name> refnum) -> (w380:T20)
      }
    }
    n171 = Select(t=Optitrack_State."Error Handling" ("OptiTrack State"), s=w337, f=w334) -> (s? t:f=w335:T14)
  }
  n172 = Merge Errors(w34, w33, w26) -> (w32:errorcluster)
  n173 = call "Release Queues.vi"("error in (no error) in"=w32, "Queues"=w28) -> ("error out"=w31:errorcluster)  [unwired: 9 in]
  n174 = call <vilib>:"Simple Error Handler.vi"("error in (no error)"=w31) -> ("error out"=w8:errorcluster)  [unwired: 4 in, 4 out]
  n175 = call "Set Controls Enable or Disable State.vi"("error in (no error)"=w8, "Refnum State"=Enabled_State_Control."Shutdown", "Refnums In"=w7) -> ()  [unwired: 8 in, 1 out]
